vi "Open.vi"(8 "error in (no error)":errorcluster, 11 "SimpleErrorLogger in":refnum<class "SimpleErrorLogger.lvclass">) -> (0 "error out":errorcluster, 3 "SimpleErrorLogger out":refnum<class "SimpleErrorLogger.lvclass">)   [LabVIEW 2023, in "SimpleErrorLogger.lvlib" / "SimpleErrorLogger.lvclass"]
uses:
  SimpleErrorLogger.lvclass
  C:/Program Files (x86)/National Instruments/LabVIEW 2023/vi.lib/ActorFramework/Actor/Actor.lvclass
  <vilib>/ActorFramework/Actor/Actor.lvclass/Actor.ctl
  <vilib>/ActorFramework/Message Enqueuer/Message Enqueuer.lvclass/Message Enqueuer.ctl
  SimpleErrorLogger.lvclass/SimpleErrorLogger.ctl
  <vilib>/ActorFramework/Message Enqueuer/Message Priority.ctl
  SimpleErrorLogger Messages/LogError Msg/LogError Msg.lvclass/LogError Msg.ctl
  <vilib>/ActorFramework/Message Enqueuer/Init from Existing Queue.vi
  <vilib>/ActorFramework/Message Enqueuer/Enqueue.vi
  SimpleErrorLogger Messages/WriteHeader Msg/WriteHeader Msg.lvclass
  C:/Program Files (x86)/National Instruments/LabVIEW 2023/vi.lib/ActorFramework/Message/Message.lvclass
  SimpleErrorLogger Messages/LogError Msg/LogError Msg.lvclass
  SimpleErrorLogger Messages/Open Msg/Open Msg.lvclass
  <vilib>/ActorFramework/Message Priority Queue/Priority Enqueue.vi
  <vilib>/ActorFramework/Message Enqueuer/Message Enqueuer.lvclass
  <vilib>/ActorFramework/Actor/Actor.lvclass
  C:/Source/LabVIEW/Error_Logger/SimpleErrorLogger/SimpleErrorLogger/SimpleErrorLogger.lvclass
  ApplicationWithErrorLogger Messages/NewErriorLoggerFile Msg/NewErriorLoggerFile Msg.lvclass
  ApplicationWithErrorLogger Messages/OpenErrorlogFileError Msg/OpenErrorlogFileError Msg.lvclass
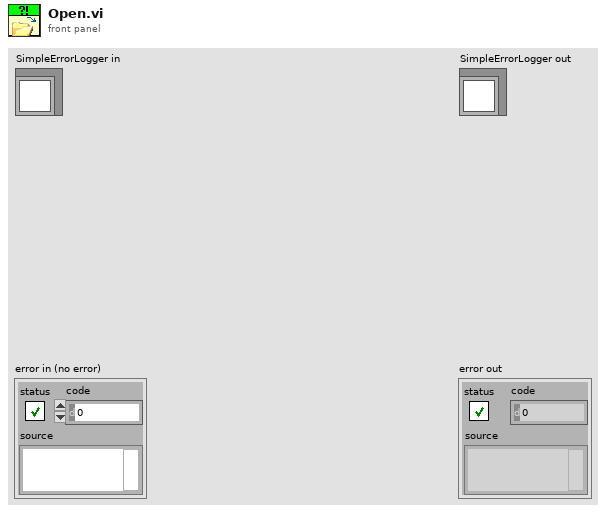
[diagram p1: front panel]
types:
  T1 = enum16{"open", "replace", "create", "open or create", "replace or create", "replace or create with confirmation"}
  T2 = typedef "Actor Framework.lvlib/Message Enqueuer.lvclass/Message Priority.ctl" = enum16{"Low", "Normal", "High"}
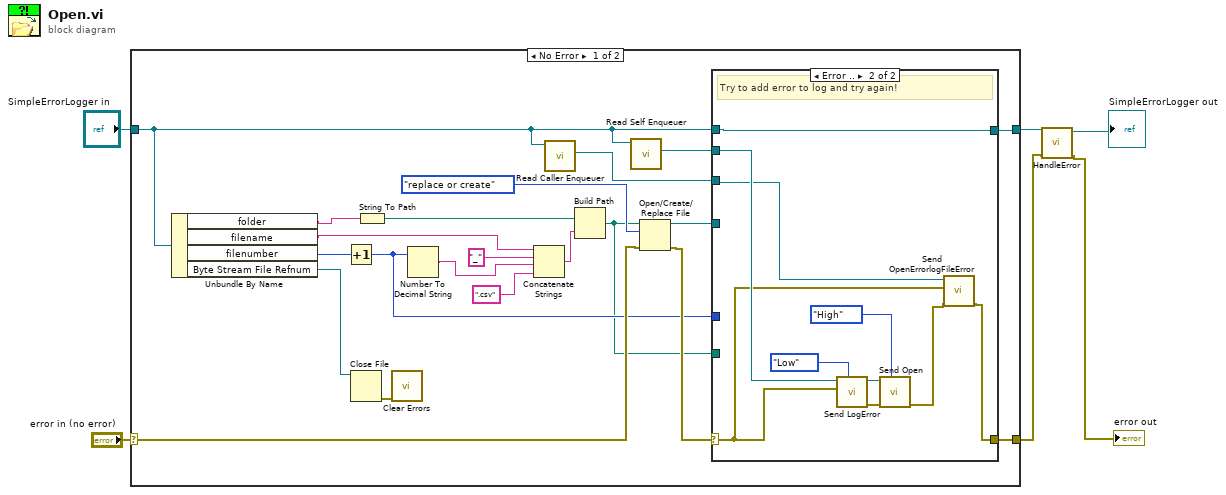
[diagram p0: block diagram]
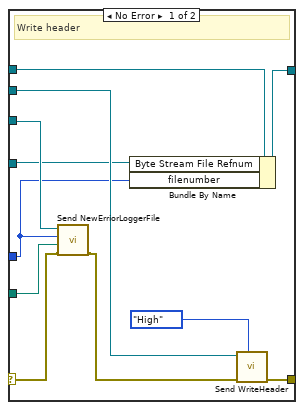
[diagram p2: hidden frame]
diagram:
  n1 = case shown="No Error" "error in (no error)" {
    selector: "error in (no error)" -> [w19 w50]
    tunnel: [w17 w50] -> w2
    tunnel: [w16 w49] -> w4
    tunnel: "SimpleErrorLogger in" -> [w9 w49]
    frame No Error {
      n2 = Unbundle By Name(w9) -> ("folder"=w26:string, "filename"=w23:string, "filenumber"=w24:u32, "Byte Stream File Refnum"=w27:refnum<file>)
      n3 = Increment(x=w24) -> (x+1=w14:u32)
      n4 = Close File(refnum=w27) -> (error out=w13:errorcluster)  [unwired: 1 in, 1 out]
      n5 = String To Path(string=w26) -> (path=w25:path)
      n6 = call <vilib>:"Clear Errors.vi"("error in (no error)"=w13) -> ()  [unwired: 5 in, 2 out]
      n7 = Number To Decimal String(number=w14) -> (decimal integer string=w21:string)  [unwired: 1 in]
      n8 = Concatenate Strings(w23, "_", w21, ".csv" ("string")) -> (w11:string)
      n9 = call <vilib>:"Read Caller Enqueuer.vi"("Actor"=w9) -> ("Caller Enqueuer"=w8:refnum<class "Message Enqueuer.lvclass">)  [unwired: 10 in]
      n10 = Build Path(base path=w25, name or relative path=w11) -> (appended path=w7:path)
      n11 = call <vilib>:"Read Self Enqueuer.vi"("Actor"=w9) -> ("Self Enqueuer"=w12:refnum<class "Message Enqueuer.lvclass">)  [unwired: 10 in]
      n12 = Open/Create/Replace File(file path (use dialog)=w7, error in=w19, operation (0:open)=T1."replace or create") -> (refnum out=w15:refnum<file>, error out=w18:errorcluster)  [unwired: 3 in, 1 out]
      n13 = case shown="Error .." w18 {
        selector: w18 -> [w29 w41]
        tunnel: [w35 w39] -> w17
        tunnel: w9 -> [w38 w48]
        tunnel: [w37 w48] -> w16
        tunnel: w15 -> [w31 _]
        tunnel: w14 -> [w32 _]
        tunnel: w12 -> [w36 w47]
        tunnel: w8 -> [w33 w42]
        tunnel: w7 -> [w30 _]
        frame No Error {
          # "Write header"
          n14 = call "Send NewErriorLoggerFile.vi"("error in (no error)"=w29, "ErrorLogPath"=w30, "Filenumber"=w32, "Message Enqueuer"=w33) -> ("error out"=w28:errorcluster)  [unwired: 6 in, 1 out]
          n15 = Bundle By Name(cluster=w38, "Byte Stream File Refnum"=w31, "filenumber"=w32) -> (w37:refnum<class "SimpleErrorLogger.lvclass">)
          n16 = call "Send WriteHeader.vi"("Message Priority (Normal)"=Message_Priority."High", "error in (no error)"=w28, "Message Enqueuer"=w36) -> ("error out"=w35:errorcluster)  [unwired: 7 in, 1 out]
        }
        frame Error {
          # "Try to add error to log and try again!"
          n17 = call "Send LogError.vi"("Message Priority (Normal)"=Message_Priority."Low", "error"=w41, "Message Enqueuer"=w47) -> ("error out"=w46:errorcluster, "Message Enqueuer out"=w45:refnum<class "Message Enqueuer.lvclass">)  [unwired: 7 in]
          n18 = call "Send Open.vi"("Message Priority (Normal)"=Message_Priority."High", "error in (no error)"=w46, "Message Enqueuer"=w45) -> ("error out"=w40:errorcluster)  [unwired: 7 in, 1 out]
          n19 = call "Send OpenErrorlogFileError.vi"("error in (no error)"=w40, "error"=w41, "Message Enqueuer"=w42) -> ("error out"=w39:errorcluster)  [unwired: 7 in, 1 out]
        }
      }
    }
    frame Error {
    }
  }
  n20 = call "HandleError.vi"("error in (no error)"=w2, "SimpleErrorLogger in"=w4) -> ("error out"=→"error out":errorcluster, "SimpleErrorLogger out"=→"SimpleErrorLogger out":refnum<class "SimpleErrorLogger.lvclass">)  [unwired: 8 in]
